vi "Get Platform Name.vi"(8 "error in (no error)":errorcluster, 11 "Device in":refnum<class "Device.lvclass">) -> (0 "error out":errorcluster, 2 "Platform":string, 3 "Device out":refnum<class "Device.lvclass">)   [LabVIEW 2020, in "PicoG-App.lvlib" / "Device.lvclass"]
uses:
  Device.lvclass
  Device.lvclass/Device.ctl
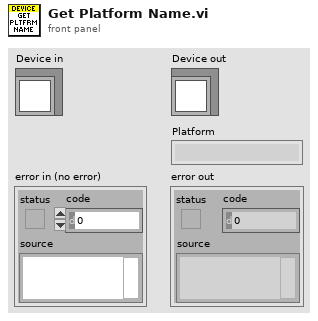
[diagram p1: front panel]
types:
  T1 = typedef "PicoG-App.lvlib/Device.lvclass/Ref Data.ctl" = cluster{"Alias":string, "Version":string, "Build":timestamp, "Key":T2}
  T2 = typedef "PicoG-App.lvlib/Device.lvclass/Device Key.ctl" = cluster{"Platform":string, "Board":string, "ID":string}
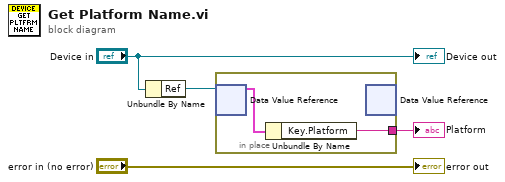
[diagram p0: block diagram]
diagram:
  n1 = Unbundle By Name("Device in") -> ("Ref"=w3:refnum<data-value>)
  n2 = in-place {
    in-place-border: [w5] -> w1
    n3 = in-place-dvr #1(w3) -> (w6:T1)  [unwired: 1 out]
    n4 = Unbundle By Name(w6) -> ("Key.Platform"=w5:string)
    n5 = in-place-dvr #1() -> ()  [unwired: 1 in, 2 out]
  }
  "Platform" <- w1
  "error out" <- "error in (no error)"
  "Device out" <- "Device in"
